vi "simflight-2.0.vi"() -> ()   [LabVIEW 2014]
uses:
  state space loop data.ctl
  <vilib>/addons/Control Design/_Model Construction/Data Typedefs.llb/CD MIMO Time Response Data.ctl
  <vilib>/addons/Control Design/_Model Construction/Data Typedefs.llb/CD Plot Types Enum.ctl
  <vilib>/Utility/miscctls.llb/LV3DPointTypeDef.ctl
  <vilib>/addons/Control Design/_Model Construction/Model Creation.llb/Model Creation SubVI/cd_Create State Space Model.vi
  <vilib>/Utility/inputDevices.llb/joystickAcquire.vi
  Data Xfer/subvis/Curcular Buffer Data History.vi
  <vilib>/addons/Control Design/_Time Response Analysis/Time Response.llb/Time Response subVI/cd_Linear Simulation (State-Space).vi
  <vilib>/addons/Control Design/_Model Construction/NI_LinSys_Model Creation.lvlib
  <vilib>/addons/Control Design/_Time Response Analysis/NI_CD_Time Response.lvlib
  <vilib>/addons/Control Design/_Model Construction/NI_LinSys_Data Typedefs.lvlib
  attitude indicator/lv-attitudecontrol.lvlib
panel:
  in  "Attitude Indicator":refnum<vi>(3d-picture)
  out "Airspeed (ft/s)":dbl(knob)=74.91519927978516 scale=0.0..120.0 scale format="%#.4f"
  out "motor (BHP)":dbl(slide) scale=-0.2..0.2
  out "altitude":T1(graph)
  out "ground track":cluster{"Time Stamp":dbl, "Data Value":dbl}[](graph)
  out "roll":dbl(slide) scale=-90.0..90.0
  out "pitch":dbl(slide) scale=-90.0..90.0
  out "rudder":dbl(slide) scale=-10.0..10.0
  out "aileron":dbl(slide) scale=-10.0..10.0
  out "elevator":dbl(slide) scale=-10.0..10.0
  out "Heading":T2(graph)={"X"=[{"Y"=[21.620706805998168, 20.15124367946963, 12.465582235692763, 7.946576972490323, 11.656565240893995, 3.970903792227472, 5.440366929130449, 13.126028372052978, 19.003880895383112, 16.244982298473555, 16.832767550897515, 24.922937499080067, 24.33515224168201, 19.81289788882929, 13.93504536742159, 21.620706805998168], "Y"=[7.099604990531346, 5.077062500919932, 10.661022401488875, 5.291796067500631, 11.248807654089271, 16.832767550897515, 18.855310035128806, 13.271350139939326, 21.36152008350073, 25.220079209877188, 26.02909620777253, 20.151243679469633, 19.34222668734553, 20.773734831883043, 12.683564887248515, 7.099604990531346]}], "z"=[{"Y"=[15.0, 16.30733614, 17.60472267, 17.43107449, 17.60472267, 18.88228568, 20.13030215, 19.78828201, 20.13030215, 21.33927393, 22.5, 22.0, 22.5, 23.60364655, 24.64181415, 23.99902654, 24.64181415, 25.60660172, 26.49066665, 25.7246222, 26.49066665, 27.28728066, 27.99038106, 27.12435565, 27.99038106, 28.59461681, 29.09538931, 28.15569669, 29.09538931, 29.48888739, 29.7721163, 28.78730854, 29.7721163, 29.94292047, 30.0, 28.5, 30.0, 29.94292047, 29.7721163, 28.78730854, 29.7721163, 29.48888739, 29.09538931, 28.15569669, 29.09538931, 28.59461681, 27.99038106, 27.12435565, 27.99038106, 27.28728066, 26.49066665, 25.7246222, 26.49066665, 25.60660172, 24.64181415, 23.99902654, 24.64181415, 23.60364655, 22.5, 22.0, 22.5, 21.33927393, 20.13030215, 19.78828201, 20.13030215, 18.88228568, 17.60472267, 17.43107449, 17.60472267, 16.30733614, 15.0, 15.0, 15.0, 13.69266386, 12.39527733, 12.56892551, 12.39527733, 11.11771432, 9.86969785, 10.21171799, 9.86969785, 8.660726074, 7.5, 8.0, 7.5, 6.396353455, 5.358185855, 6.000973464, 5.358185855, 4.393398282, 3.509333353, 4.275377796, 3.509333353, 2.712719336, 2.009618943, 2.875644347, 2.009618943, 1.405383194, 0.904610688, 1.844303309, 0.904610688, 0.511112606, 0.227883705, 1.212691458, 0.227883705, 0.057079529, 0.0, 1.5, 0.0, 0.057079529, 0.227883705, 1.212691458, 0.227883705, 0.511112606, 0.904610688, 1.844303309, 0.904610688, 1.405383194, 2.009618943, 2.875644347, 2.009618943, 2.712719336, 3.509333353, 4.275377796, 3.509333353, 4.393398282, 5.358185855, 6.000973464, 5.358185855, 6.396353455, 7.5, 8.0, 7.5, 8.660726074, 9.86969785, 10.21171799, 9.86969785, 11.11771432, 12.39527733, 12.56892551, 12.39527733, 13.69266386, 15.0, 15.0], "Y"=[30.0, 29.94292047, 29.7721163, 28.78730854, 29.7721163, 29.48888739, 29.09538931, 28.15569669, 29.09538931, 28.59461681, 27.99038106, 27.12435565, 27.99038106, 27.28728066, 26.49066665, 25.7246222, 26.49066665, 25.60660172, 24.64181415, 23.99902654, 24.64181415, 23.60364655, 22.5, 22.0, 22.5, 21.33927393, 20.13030215, 19.78828201, 20.13030215, 18.88228568, 17.60472267, 17.43107449, 17.60472267, 16.30733614, 15.0, 15.0, 15.0, 13.69266386, 12.39527733, 12.56892551, 12.39527733, 11.11771432, 9.86969785, 10.21171799, 9.86969785, 8.660726074, 7.5, 8.0, 7.5, 6.396353455, 5.358185855, 6.000973464, 5.358185855, 4.393398282, 3.509333353, 4.275377796, 3.509333353, 2.712719336, 2.009618943, 2.875644347, 2.009618943, 1.405383194, 0.904610688, 1.844303309, 0.904610688, 0.511112606, 0.227883705, 1.212691458, 0.227883705, 0.057079529, 0.0, 1.5, 0.0, 0.057079529, 0.227883705, 1.212691458, 0.227883705, 0.511112606, 0.904610688, 1.844303309, 0.904610688, 1.405383194, 2.009618943, 2.875644347, 2.009618943, 2.712719336, 3.509333353, 4.275377796, 3.509333353, 4.393398282, 5.358185855, 6.000973464, 5.358185855, 6.396353455, 7.5, 8.0, 7.5, 8.660726074, 9.86969785, 10.21171799, 9.86969785, 11.11771432, 12.39527733, 12.56892551, 12.39527733, 13.69266386, 15.0, 15.0, 15.0, 16.30733614, 17.60472267, 17.43107449, 17.60472267, 18.88228568, 20.13030215, 19.78828201, 20.13030215, 21.33927393, 22.5, 22.0, 22.5, 23.60364655, 24.64181415, 23.99902654, 24.64181415, 25.60660172, 26.49066665, 25.7246222, 26.49066665, 27.28728066, 27.99038106, 27.12435565, 27.99038106, 28.59461681, 29.09538931, 28.15569669, 29.09538931, 29.48888739, 29.7721163, 28.78730854, 29.7721163, 29.94292047, 30.0, 28.5]}]}
  in  "visual":refnum<k7>(container) caption="3D 파라미터형 표면"
  in  "stop":bool
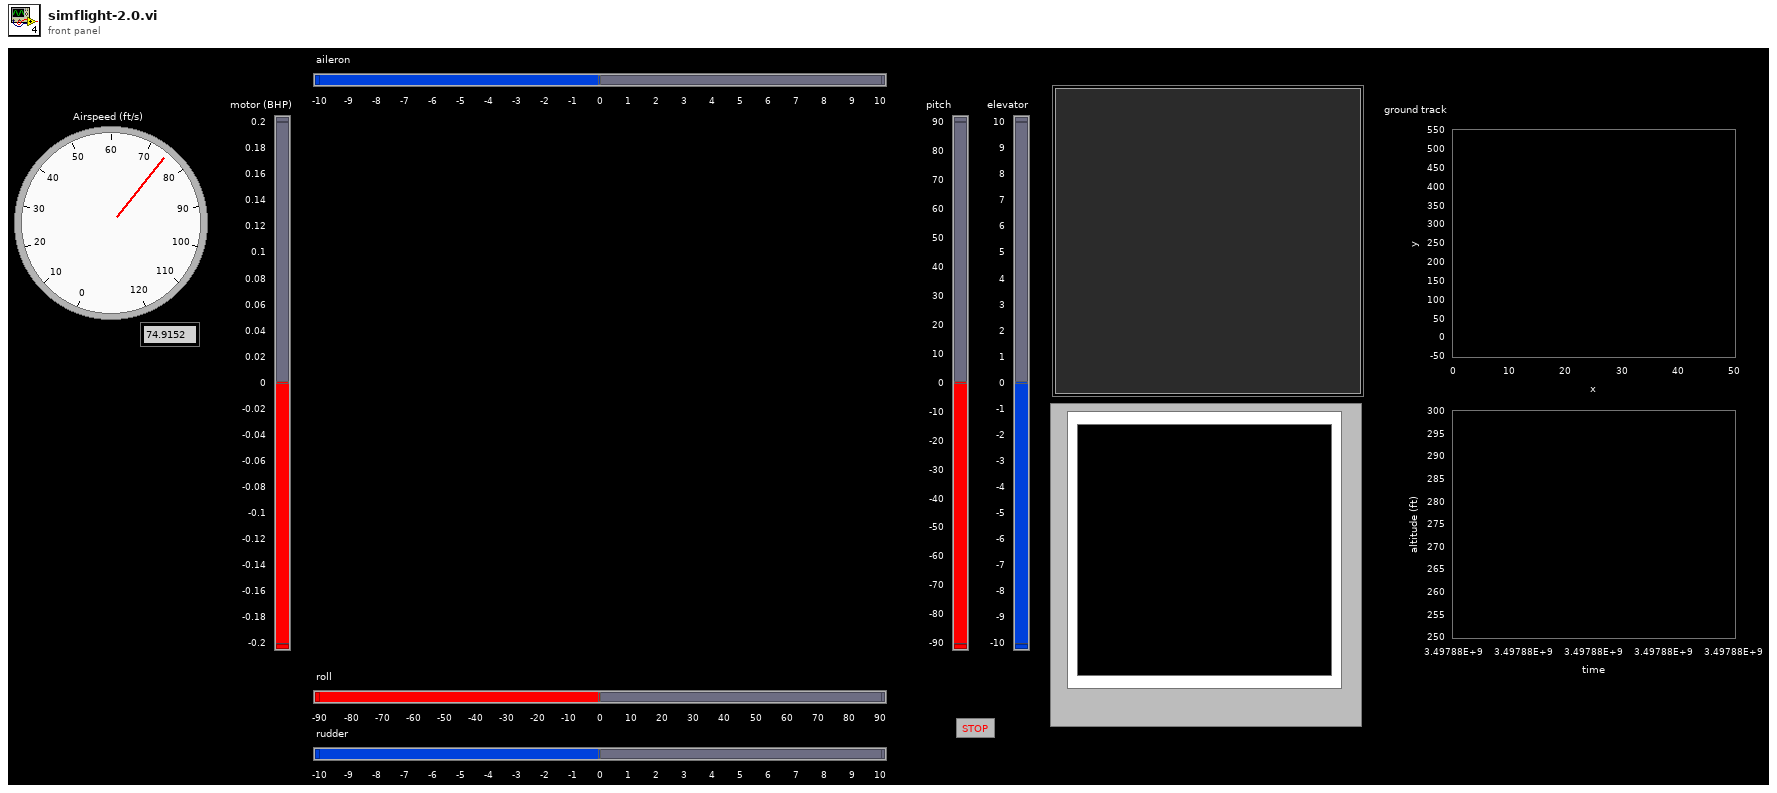
[diagram p1: front panel]
types:
  T1 = cluster{cluster{"Time Stamp":dbl, "Data Value":dbl}[]}[]
  T2 = cluster{"X":cluster{"Y":dbl[], "Y":dbl[]}[], "z":cluster{"Y":dbl[], "Y":dbl[]}[]}
  T3 = typedef "state space loop data.ctl" = cluster{"d_elevator (rad)":dbl, "d_rudder (rad)":dbl, "d_aileron (rad)":dbl, "d_motor (bhp)":dbl, "loop start (s)":dbl, "dT":dbl, "time now":dbl, "Sim Data":T4, "sim conditions":dbl[], "timestamp":dbl}
  T4 = typedef "NI_LinSys_Data Typedefs.lvlib/CD MIMO Time Response Data.ctl" = cluster{"Time":dbl[], "Outputs Data":dbl[][][], "States Data":dbl[][][], "plot type":T5}
  T5 = typedef "NI_LinSys_Data Typedefs.lvlib/CD Plot Types Enum.ctl" = enum16{"bode-magnitude", "bode-phase", "nichols", "nyquist", "singular values", "step", "impulse", "initial", "simulation", "nyquist with separation"}
  T6 = typedef "NI_LinSys_Model Typedefs.lvlib/CD State Space Model (MIMO).ctl" = cluster{"properties":T7, "A":dbl[][], "B":dbl[][], "C":dbl[][], "D":dbl[][], "StateNames":string[], "Transport Delay":dbl[][]}
  T7 = typedef "NI_LinSys_Model Typedefs.lvlib/CD General Elements.ctl" = cluster{"Model name":string, "Input names":string[], "Output names":string[], "Input Delays":dbl[], "Output Delays":dbl[], "Sampling Time":dbl, "Notes":string}
  T8 = typedef "lv-attitudecontrol.lvlib/AttitudeHandle.ctl" = cluster{"First Scene Object":refnum<vi>, "Drum":refnum<vi>, "Window":refnum<vi>, "Dial":refnum<vi>, "Scene Graph":refnum<vi>, "Last Drum Pitch":dbl, "Last Drum Roll ":dbl, "Last Dial Roll":dbl}
  T9 = cluster{"X axis":i32, "Y axis":i32, "Z axis":i32, "X axis rotation":i32, "Y axis rotation":i32, "Z axis rotation":i32, "U axis":i32, "V axis":i32}
  T10 = typedef "LV3DPointTypeDef.ctl" = cluster{"X":sgl, "Y":sgl, "Z":sgl}
  T11 = cluster{cluster{"Time Stamp":dbl, "Data Value":dbl}[]}
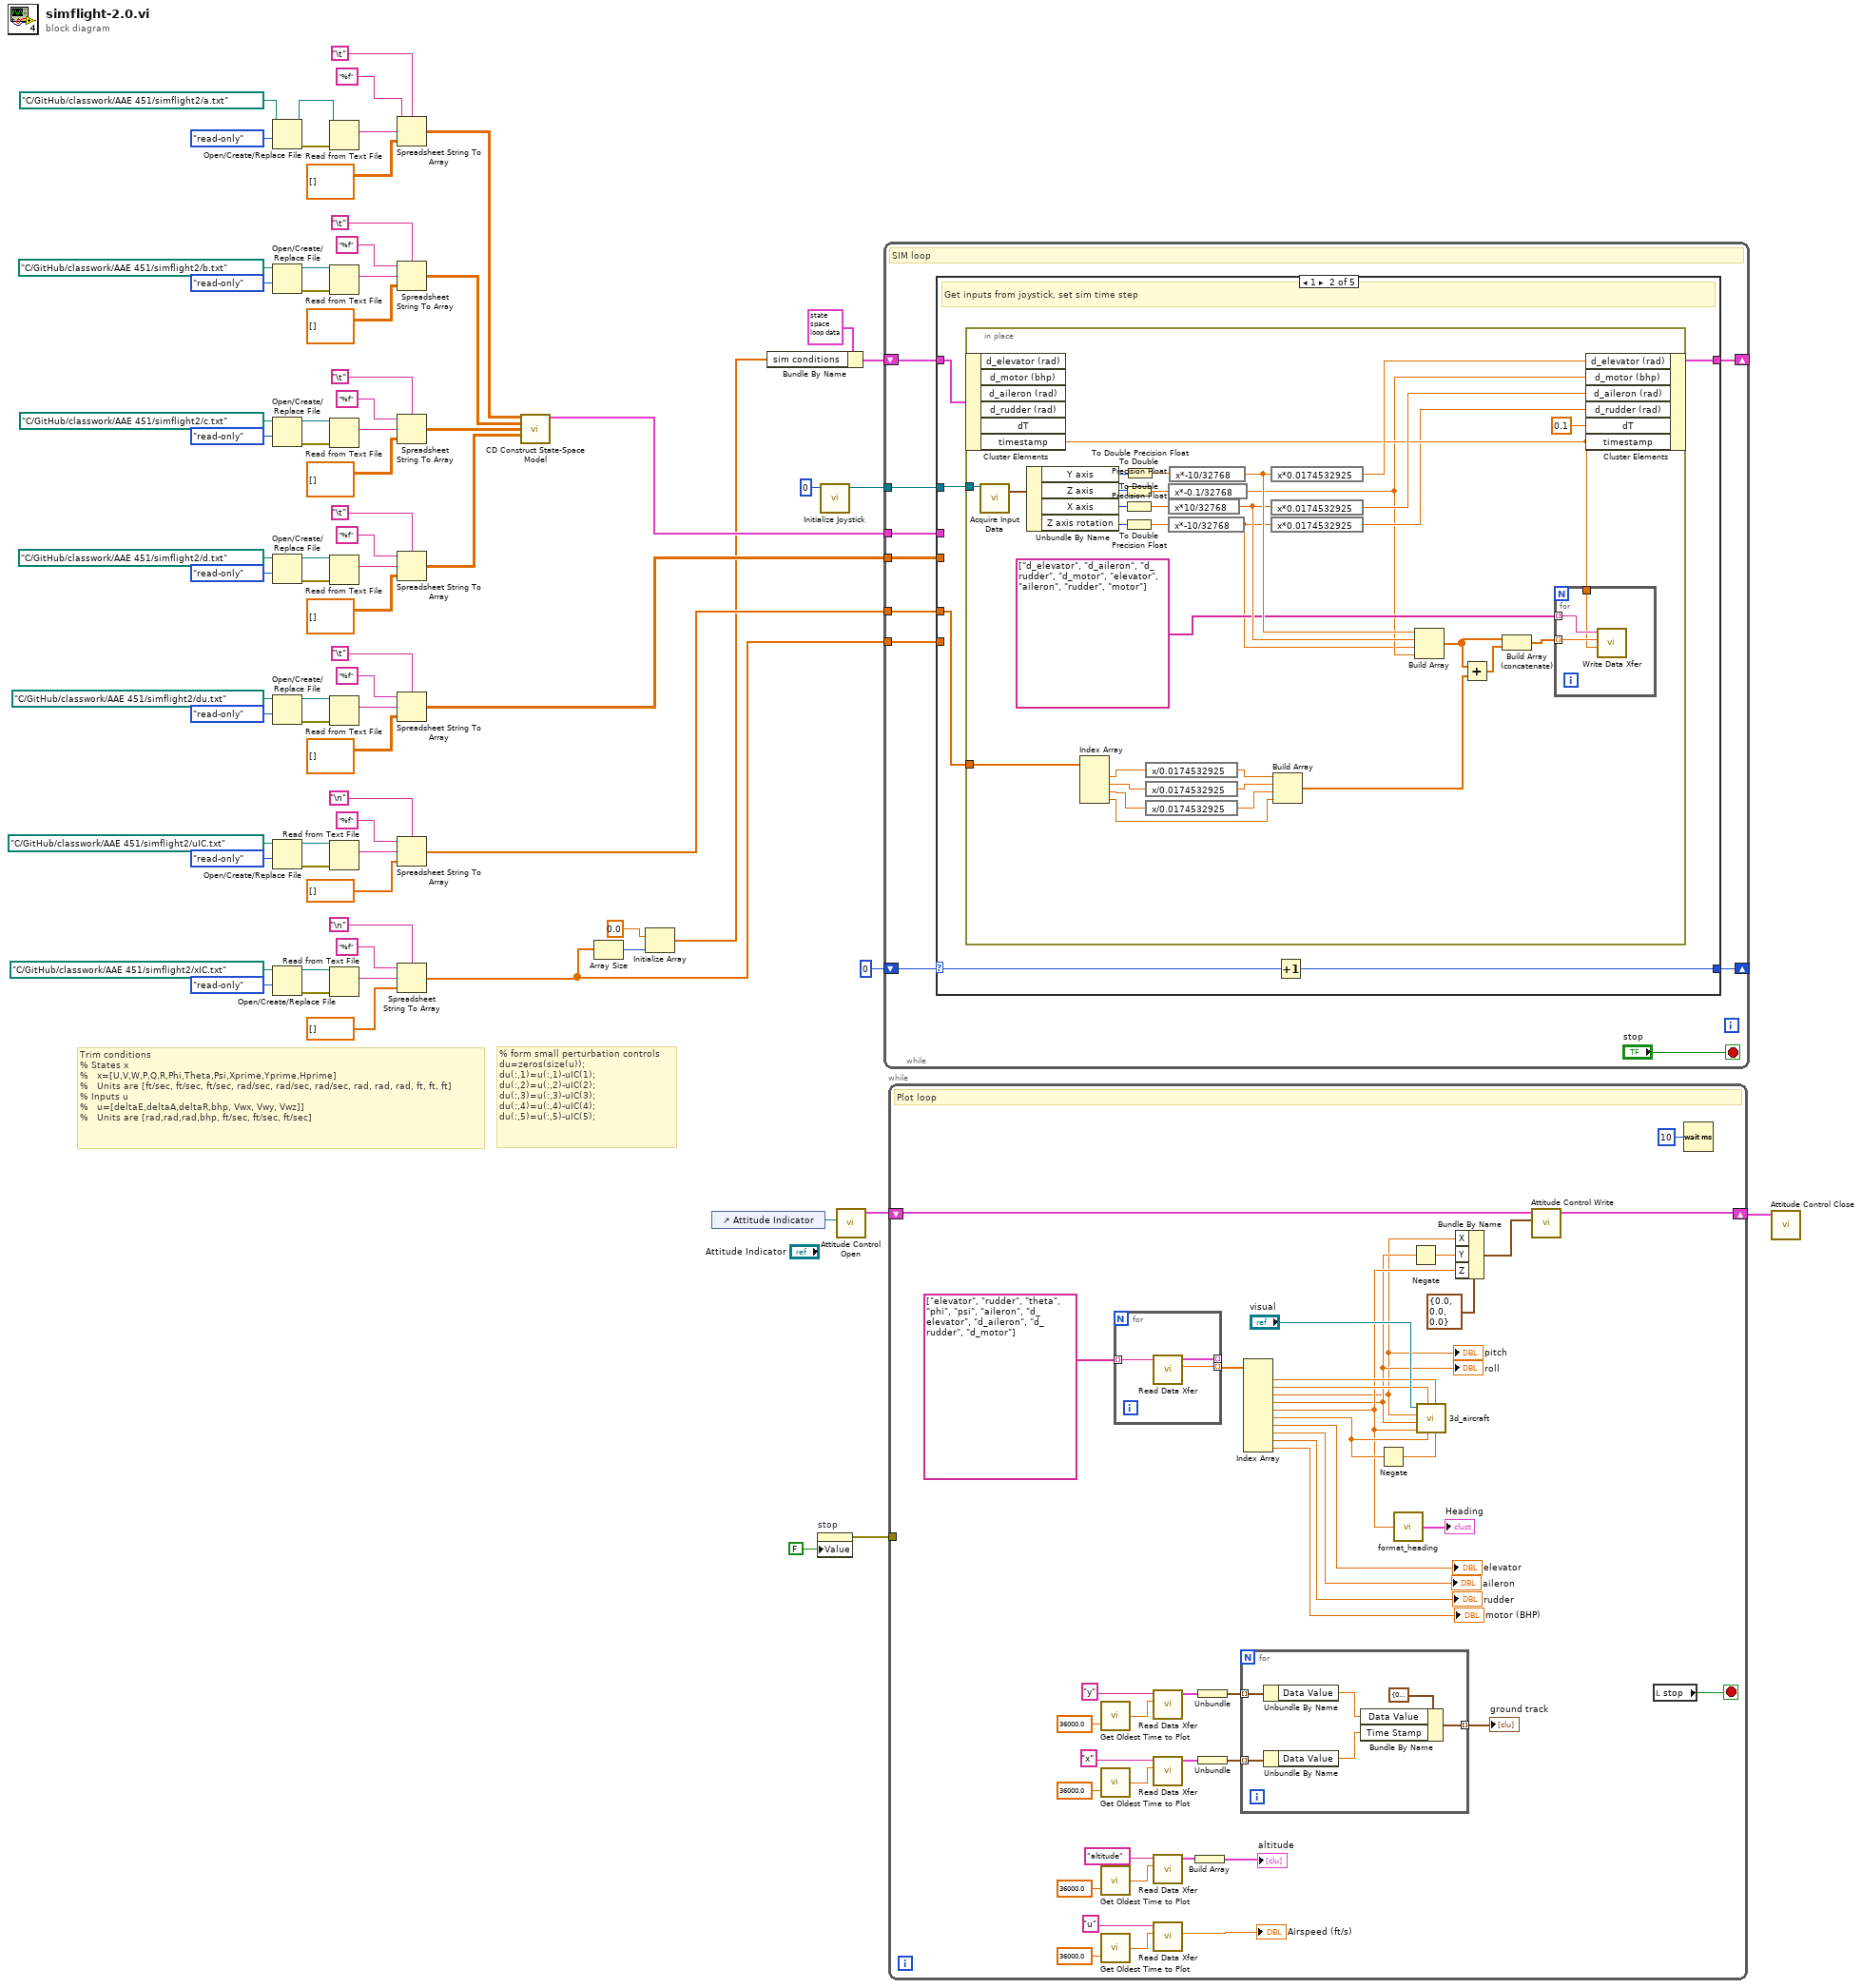
[diagram p0: block diagram]
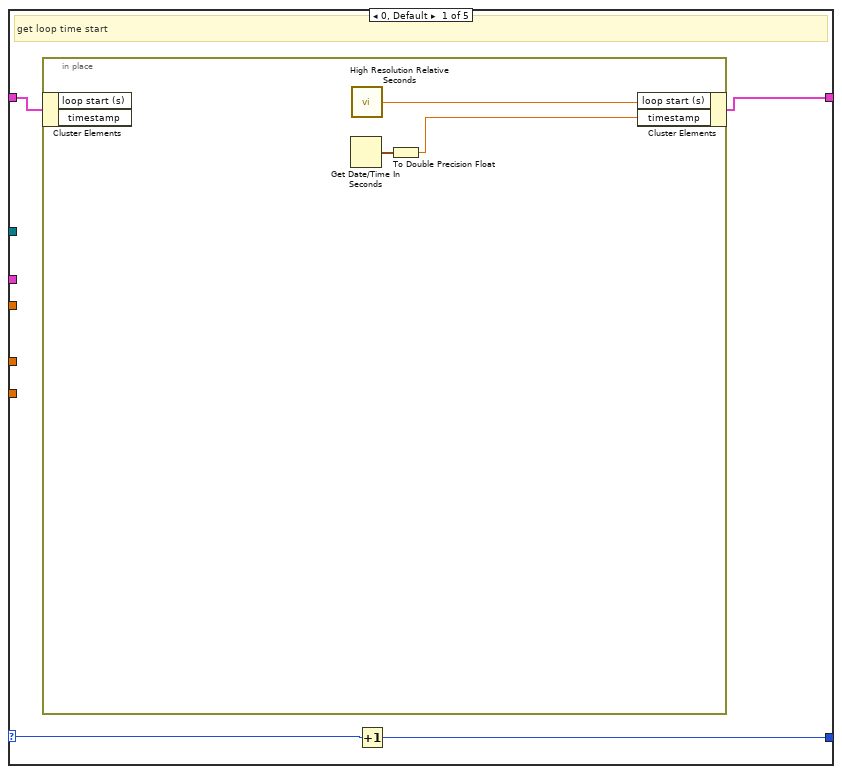
[diagram p2: hidden frame]
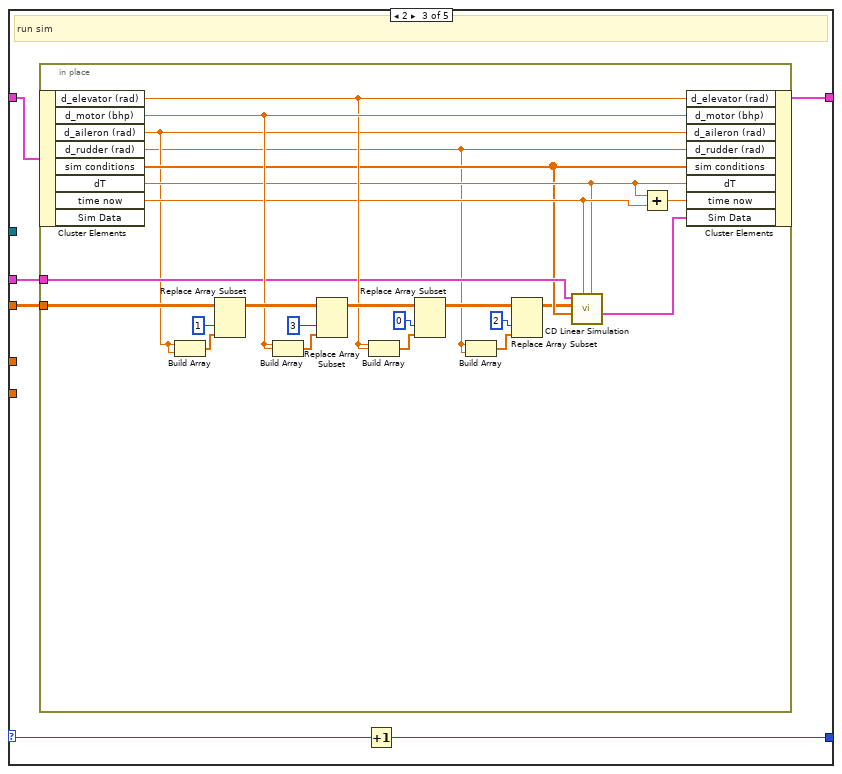
[diagram p3: hidden frame]
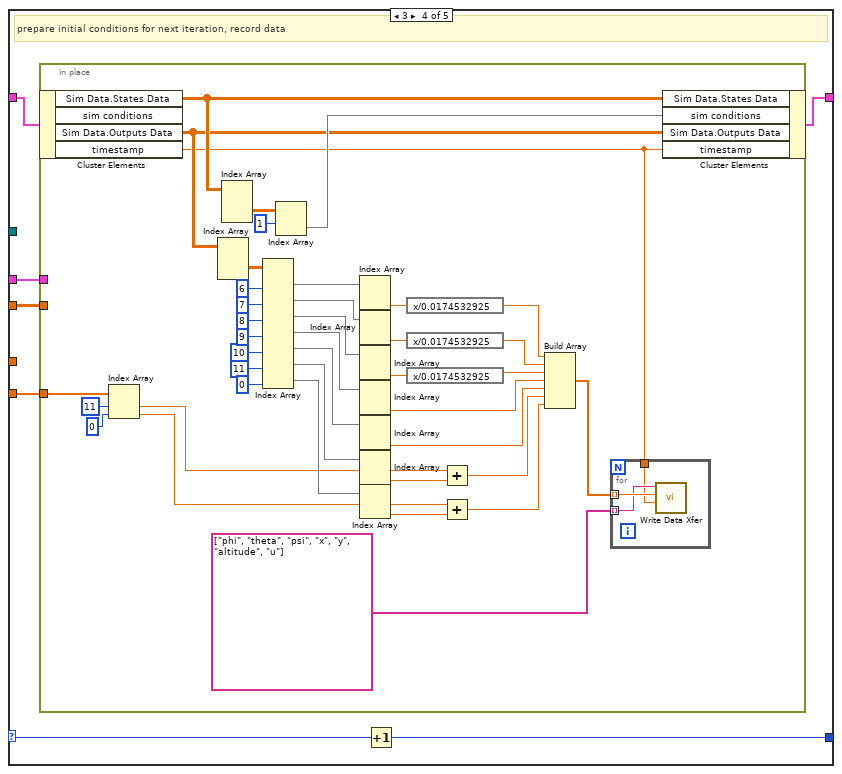
[diagram p4: hidden frame]
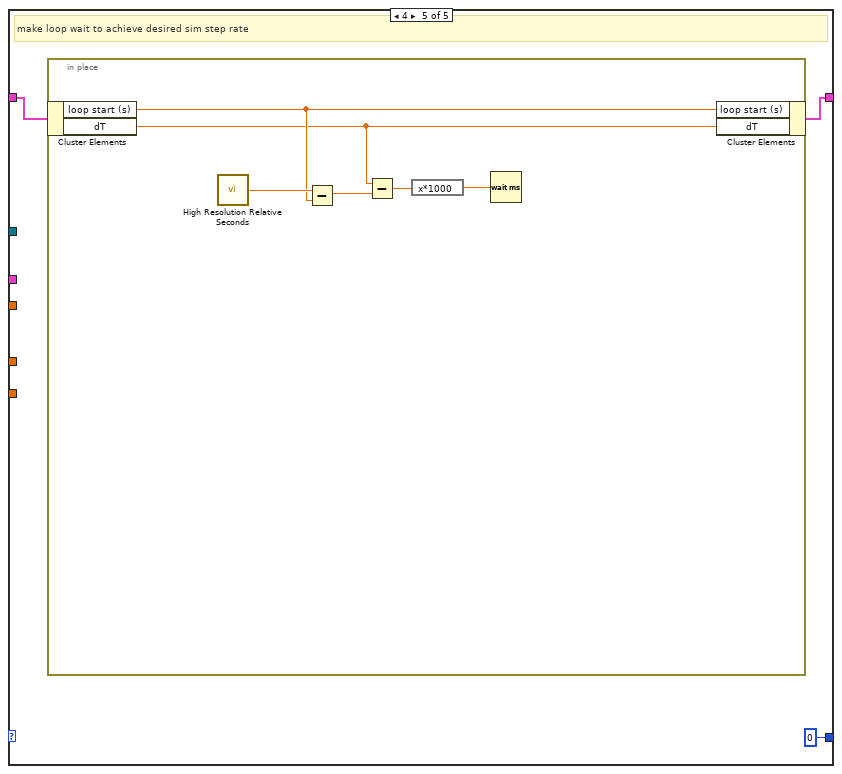
[diagram p5: hidden frame]
diagram:
  # "% form small perturbation controls\ndu=zeros(size(u));\ndu(:,1)=u(:,1)-uIC(1);\ndu(:,2)=u(:,2)-uIC(2);\ndu(:,3)=u(:,3)-uIC(3);\ndu(:,4)=u(:,4)-uIC(4);\ndu(:,5)=u(:,5)-uIC(5);"
  # "Trim conditions\n% States x\n%   x=[U,V,W,P,Q,R,Phi,Theta,Psi,Xprime,Yprime,Hprime]\n%   Units are [ft/sec, ft/sec, ft/sec, rad/sec, rad/sec, rad/sec, rad, rad, rad, ft, ft, ft]\n% Inputs u\n%   u=[deltaE,deltaA,deltaR,bhp, Vwx, Vwy, Vwz]]\n%   Units are [rad,rad,rad,bhp, ft/sec, ft/sec, ft/sec]"
  n1 = Open/Create/Replace File(file path (use dialog)=path "C:/GitHub/classwork/AAE 451/simflight2/a.txt", access (0:read/write)=enum16{"read/write", "read-only", "write-only"}."read-only") -> (refnum out=w74:refnum<file>, error out=w75:errorcluster)  [unwired: 4 in, 1 out]
  n2 = Open/Create/Replace File(file path (use dialog)=path "C:/GitHub/classwork/AAE 451/simflight2/b.txt", access (0:read/write)=enum16{"read/write", "read-only", "write-only"}."read-only") -> (refnum out=w65:refnum<file>, error out=w64:errorcluster)  [unwired: 4 in, 1 out]
  n3 = Open/Create/Replace File(file path (use dialog)=path "C:/GitHub/classwork/AAE 451/simflight2/c.txt", access (0:read/write)=enum16{"read/write", "read-only", "write-only"}."read-only") -> (refnum out=w58:refnum<file>, error out=w59:errorcluster)  [unwired: 4 in, 1 out]
  n4 = Open/Create/Replace File(file path (use dialog)=path "C:/GitHub/classwork/AAE 451/simflight2/d.txt", access (0:read/write)=enum16{"read/write", "read-only", "write-only"}."read-only") -> (refnum out=w49:refnum<file>, error out=w48:errorcluster)  [unwired: 4 in, 1 out]
  n5 = Open/Create/Replace File(file path (use dialog)=path "C:/GitHub/classwork/AAE 451/simflight2/du.txt", access (0:read/write)=enum16{"read/write", "read-only", "write-only"}."read-only") -> (refnum out=w38:refnum<file>, error out=w39:errorcluster)  [unwired: 4 in, 1 out]
  n6 = Open/Create/Replace File(file path (use dialog)=path "C:/GitHub/classwork/AAE 451/simflight2/uIC.txt", access (0:read/write)=enum16{"read/write", "read-only", "write-only"}."read-only") -> (refnum out=w15:refnum<file>, error out=w16:errorcluster)  [unwired: 4 in, 1 out]
  n7 = Open/Create/Replace File(file path (use dialog)=path "C:/GitHub/classwork/AAE 451/simflight2/xIC.txt", access (0:read/write)=enum16{"read/write", "read-only", "write-only"}."read-only") -> (refnum out=w30:refnum<file>, error out=w31:errorcluster)  [unwired: 4 in, 1 out]
  n8 = Read from Text File(file (use dialog)=w74, error in=w75) -> (text=w73:string)  [unwired: 2 in, 3 out]
  n9 = Read from Text File(file (use dialog)=w65, error in=w64) -> (text=w66:string)  [unwired: 2 in, 3 out]
  n10 = Read from Text File(file (use dialog)=w58, error in=w59) -> (text=w57:string)  [unwired: 2 in, 3 out]
  n11 = Read from Text File(file (use dialog)=w49, error in=w48) -> (text=w50:string)  [unwired: 2 in, 3 out]
  n12 = Read from Text File(file (use dialog)=w38, error in=w39) -> (text=w37:string)  [unwired: 2 in, 3 out]
  n13 = Read from Text File(file (use dialog)=w15, error in=w16) -> (text=w14:string)  [unwired: 2 in, 3 out]
  n14 = Read from Text File(file (use dialog)=w30, error in=w31) -> (text=w29:string)  [unwired: 2 in, 3 out]
  n15 = Spreadsheet String To Array(delimiter (Tab)="\t", format string="%f", spreadsheet string=w73, array type (2D Dbl)=dbl[][] []) -> (array=w45:dbl[][])
  n16 = Spreadsheet String To Array(delimiter (Tab)="\t", format string="%f", spreadsheet string=w66, array type (2D Dbl)=dbl[][] []) -> (array=w44:dbl[][])
  n17 = Spreadsheet String To Array(delimiter (Tab)="\t", format string="%f", spreadsheet string=w57, array type (2D Dbl)=dbl[][] []) -> (array=w42:dbl[][])
  n18 = Spreadsheet String To Array(delimiter (Tab)="\t", format string="%f", spreadsheet string=w50, array type (2D Dbl)=dbl[][] []) -> (array=w43:dbl[][])
  n19 = Spreadsheet String To Array(delimiter (Tab)="\t", format string="%f", spreadsheet string=w37, array type (2D Dbl)=dbl[][] []) -> (array=w21:dbl[][])
  n20 = Spreadsheet String To Array(delimiter (Tab)="\n", format string="%f", spreadsheet string=w14, array type (2D Dbl)=dbl[] []) -> (array=w10:dbl[])
  n21 = Spreadsheet String To Array(delimiter (Tab)="\n", format string="%f", spreadsheet string=w29, array type (2D Dbl)=dbl[] []) -> (array=w4:dbl[])
  n22 = call-poly <vilib>:"CD Construct State-Space Model.vi"("A"=w45, "B"=w44, "C"=w42, "D"=w43) -> ("State-Space Model"=w22:T6)  [unwired: 10 in, 1 out]
  n23 = Array Size(array=w4) -> (size(s)=w7:i32)
  n24 = Initialize Array(0.0, w7) -> (w5:dbl[])
  n25 = control-ref of="Attitude Indicator"() -> (w3:refnum<vi>)
  n26 = Bundle By Name(cluster=T3 {"d_elevator (rad)"=0.0, "d_rudder (rad)"=0.0, "d_aileron (rad)"=0.0, "d_motor (bhp)"=0.0, "loop start (s)"=0.0, "dT"=0.0, "time now"=0.0, "Sim Data"={"Time"=[], "Outputs Data"=[], "States Data"=[], "plot type"=enum."step"}, "sim conditions"=[], "timestamp"=0.0}, "sim conditions"=w5) -> (w19:T3)
  n27 = property on="stop" class="Bool (strict)"("Value"=FALSE ("stop")) -> (error out=w8:errorcluster)  [unwired: 2 in, 1 out]
  n28 = call <vilib>:"Initialize Joystick.vi"("device index"=0) -> ("device ID"=w24:refnum<k1>)  [unwired: 9 in, 1 out]
  n29 = call "Attitude Control Open.vi"("Scene Graph"=w3) -> ("Attitude Control Handle"=w2:T8)  [unwired: 9 in, 1 out]
  n30 = while {
    shift-right: [w86] -> _
    shift-left: w19 -> [w87]
    tunnel: w24 -> [w85]
    shift-right: [w84] -> _
    shift-left: 0 -> [w83]
    tunnel: w22 -> [w81]
    tunnel: w21 -> [w80]
    tunnel: w10 -> [w79]
    tunnel: w4 -> [w78]
    stop <- "stop" stop-if-true
    # "SIM loop"
    n31 = case shown="1" w83 {
      tunnel: w87 -> [w89 w99 w141 w171 w216]
      tunnel: [w88 w98 w140 w170 w215] -> w86
      tunnel: w85 -> [_ w100 _ _ _]
      selector: w83 -> [w91 w97 w139 w169 _]
      tunnel: [w90 w96 w138 w168 0] -> w84
      tunnel: w81 -> [_ _ w136 w166 _]
      tunnel: w80 -> [_ _ w137 w167 _]
      tunnel: w79 -> [_ w95 _ _ _]
      tunnel: w78 -> [_ _ _ w165 _]
      frame 0, Default {
        # "get loop time start"
        n32 = in-place {
          n33 = in-place-cluster #1(w89) -> ()  [unwired: 2 out]
          n34 = Get Date/Time In Seconds() -> (seconds since 1Jan1904=w93:timestamp)
          n35 = call <vilib>:"High Resolution Relative Seconds.vi"() -> ("relative seconds"=w94:dbl)
          n36 = To Double Precision Float(number=w93) -> (double precision float=w92:dbl)
          n37 = in-place-cluster #1("loop start (s)"=w94, "timestamp"=w92) -> (w88:T3)
        }
        n38 = Increment(x=w91) -> (x+1=w90:i32)
      }
      frame 1 {
        # "Get inputs from joystick, set sim time step"
        n39 = in-place {
          in-place-border: w100 -> [w130]
          in-place-border: w95 -> [w118]
          n40 = in-place-cluster #2(w99) -> ("timestamp"=w119:dbl)  [unwired: 5 out]
          n41 = call-poly <vilib>:"Acquire Input Data.vi"("device ID"=w130) -> ("axis info"=w129:T9)  [unwired: 14 in, 4 out]
          n42 = Unbundle By Name(w129) -> ("Y axis"=w131:i32, "Z axis"=w126:i32, "X axis"=w125:i32, "Z axis rotation"=w108:i32)
          n43 = Index Array(array=w118) -> (element #1=w113:dbl, element #2=w111:dbl, element #3=w103:dbl, element #4=w101:dbl)  [unwired: 4 in]
          n44 = To Double Precision Float(number=w126) -> (double precision float=w127:dbl)
          n45 = To Double Precision Float(number=w125) -> (double precision float=w109:dbl)
          n46 = To Double Precision Float(number=w108) -> (double precision float=w107:dbl)
          n47 = To Double Precision Float(number=w131) -> (double precision float=w132:dbl)
          n48 = expression code="x/0.0174532925"(w113) -> (w112:dbl)
          n49 = expression code="x/0.0174532925"(w111) -> (w110:dbl)
          n50 = expression code="x/0.0174532925"(w103) -> (w102:dbl)
          n51 = expression code="x*-0.1/32768"(w127) -> (w105:dbl)
          n52 = expression code="x*10/32768"(w109) -> (w121:dbl)
          n53 = expression code="x*-10/32768"(w107) -> (w104:dbl)
          n54 = expression code="x*-10/32768"(w132) -> (w122:dbl)
          n55 = expression code="x*0.0174532925"(w122) -> (w128:dbl)
          n56 = expression code="x*0.0174532925"(w121) -> (w124:dbl)
          n57 = expression code="x*0.0174532925"(w104) -> (w106:dbl)
          n58 = Build Array(w112, w110, w102, w101) -> (w117:dbl[])
          n59 = Build Array(w122, w121, w104, w105) -> (w115:dbl[])
          n60 = Add(x=w115, y=w117) -> (x+y=w116:dbl[])
          n61 = Build Array (concatenate)(w115, w116) -> (w114:dbl[])
          n62 = for {
            tunnel: w114 -> [w135] mode=indexing
            tunnel: string[] ["d_elevator", "d_aileron", "d_rudder", "d_motor", "elevator", "aileron", "rudder", "motor"] -> [w134] mode=indexing
            tunnel: w119 -> [w133]
            n63 = call "Write Data Xfer.vi"("Time Stamp"=w133, "Data Value"=w135, "Device Name"=w134) -> ()  [unwired: 8 in, 1 out]
          }
          n64 = in-place-cluster #2("d_elevator (rad)"=w128, "d_motor (bhp)"=w105, "d_aileron (rad)"=w124, "d_rudder (rad)"=w106, "dT"=0.1, "timestamp"=w119) -> (w98:T3)
        }
        n65 = Increment(x=w97) -> (x+1=w96:i32)
      }
      frame 2 {
        # "run sim"
        n66 = in-place {
          in-place-border: w137 -> [w159]
          in-place-border: w136 -> [w153]
          n67 = in-place-cluster #3(w141) -> ("d_elevator (rad)"=w154:dbl, "d_motor (bhp)"=w156:dbl, "d_aileron (rad)"=w147:dbl, "d_rudder (rad)"=w142:dbl, "sim conditions"=w148:dbl[], "dT"=w151:dbl, "time now"=w152:dbl)  [unwired: 1 out]
          n68 = Build Array(w147, w147) -> (w158:dbl[])
          n69 = Replace Array Subset(array=w159, new element=w158, index (col)=1 ("disabled index (col)")) -> (w164:dbl[][])  [unwired: 1 in]
          n70 = Build Array(w156, w156) -> (w157:dbl[])
          n71 = Replace Array Subset(array=w164, new element=w157, index (col)=3 ("disabled index (col)")) -> (w161:dbl[][])  [unwired: 1 in]
          n72 = Build Array(w154, w154) -> (w155:dbl[])
          n73 = Replace Array Subset(array=w161, new element=w155, index (col)=0 ("index")) -> (w144:dbl[][])  [unwired: 1 in]
          n74 = Build Array(w142, w142) -> (w146:dbl[])
          n75 = Replace Array Subset(array=w144, new element=w146, index (col)=2 ("index")) -> (w143:dbl[][])  [unwired: 1 in]
          n76 = call-poly <vilib>:"CD Linear Simulation.vi"("Delta t"=w151, "Initial Time"=w152, "Initial Conditions"=w148, "Inputs"=w143, "State-Space Model"=w153) -> ("Simulation Data"=w149:T4)  [unwired: 3 in, 3 out]
          n77 = Add(x=w151, y=w152) -> (x+y=w150:dbl)
          n78 = in-place-cluster #3("d_elevator (rad)"=w154, "d_motor (bhp)"=w156, "d_aileron (rad)"=w147, "d_rudder (rad)"=w142, "sim conditions"=w148, "dT"=w151, "time now"=w150, "Sim Data"=w149) -> (w140:T3)
        }
        n79 = Increment(x=w139) -> (x+1=w138:i32)
      }
      frame 3 {
        # "prepare initial conditions for next iteration, record data"
        n80 = in-place {
          in-place-border: w167 -> [_]
          in-place-border: w166 -> [_]
          in-place-border: w165 -> [w180]
          n81 = in-place-cluster #4(w171) -> ("Sim Data.States Data"=w209:dbl[][][], "Sim Data.Outputs Data"=w207:dbl[][][], "timestamp"=w190:dbl)  [unwired: 1 out]
          n82 = Index Array(array=w180, index #1=11 ("index"), index #2=0 ("index")) -> (element #1=w178:dbl, element #2=w173:dbl)
          n83 = Index Array(array=w207) -> (element=w206:dbl[][])  [unwired: 3 in]
          n84 = Index Array(array=w209) -> (element=w210:dbl[][])  [unwired: 3 in]
          n85 = Index Array(array=w206, index (col) #1=6 ("disabled index (col)"), index (col) #2=7 ("disabled index (col)"), index (col) #3=8 ("disabled index (col)"), index (col) #4=9 ("disabled index (col)"), index (col) #5=10 ("disabled index (col)"), index (col) #6=11 ("disabled index (col)"), index (col) #7=0 ("disabled index (col)")) -> (element #1=w204:dbl[], element #2=w203:dbl[], element #3=w202:dbl[], element #4=w201:dbl[], element #5=w200:dbl[], element #6=w199:dbl[], element #7=w181:dbl[])  [unwired: 7 in]
          n86 = Index Array(array=w210, index (row)=1) -> (element=w208:dbl[])  [unwired: 1 in]
          n87 = Index Array(array=w204) -> (element #2=w198:dbl)  [unwired: 2 in, 1 out]
          n88 = Index Array(array=w203) -> (element #2=w195:dbl)  [unwired: 2 in, 1 out]
          n89 = Index Array(array=w202) -> (element #2=w194:dbl)  [unwired: 2 in, 1 out]
          n90 = Index Array(array=w201) -> (element #2=w186:dbl)  [unwired: 2 in, 1 out]
          n91 = Index Array(array=w200) -> (element #2=w185:dbl)  [unwired: 2 in, 1 out]
          n92 = Index Array(array=w199) -> (element #2=w179:dbl)  [unwired: 2 in, 1 out]
          n93 = Index Array(array=w181) -> (element #2=w174:dbl)  [unwired: 2 in, 1 out]
          n94 = expression code="x/0.0174532925"(w198) -> (w189:dbl)
          n95 = expression code="x/0.0174532925"(w195) -> (w188:dbl)
          n96 = expression code="x/0.0174532925"(w194) -> (w187:dbl)
          n97 = Add(x=w178, y=w179) -> (x+y=w175:dbl)
          n98 = Add(x=w173, y=w174) -> (x+y=w172:dbl)
          n99 = Build Array(w189, w188, w187, w186, w185, w175, w172) -> (w184:dbl[])
          n100 = for {
            tunnel: w184 -> [w214] mode=indexing
            tunnel: string[] ["phi", "theta", "psi", "x", "y", "altitude", "u"] -> [w213] mode=indexing
            tunnel: w190 -> [w212]
            n101 = call "Write Data Xfer.vi"("Time Stamp"=w212, "Data Value"=w214, "Device Name"=w213) -> ()  [unwired: 8 in, 1 out]
          }
          n102 = in-place-cluster #4("Sim Data.States Data"=w209, "sim conditions"=w208, "Sim Data.Outputs Data"=w207, "timestamp"=w190) -> (w170:T3)
        }
        n103 = Increment(x=w169) -> (x+1=w168:i32)
      }
      frame 4 {
        # "make loop wait to achieve desired sim step rate"
        n104 = in-place {
          n105 = in-place-cluster #5(w216) -> ("loop start (s)"=w221:dbl, "dT"=w220:dbl)
          n106 = call <vilib>:"High Resolution Relative Seconds.vi"() -> ("relative seconds"=w223:dbl)
          n107 = Subtract(x=w223, y=w221) -> (x-y=w222:dbl)
          n108 = Subtract(x=w220, y=w222) -> (x-y=w218:dbl)
          n109 = expression code="x*1000"(w218) -> (w219:dbl)
          n110 = Wait (ms)(milliseconds to wait=w219) -> ()  [unwired: 1 out]
          n111 = in-place-cluster #5("loop start (s)"=w221, "dT"=w220) -> (w215:T3)
        }
      }
    }
  }
  n112 = while {
    tunnel: w8 -> [_]
    shift-right: [w227] -> w1
    shift-left: w2 -> [w229]
    stop <- w265 stop-if-true
    # "Plot loop"
    n113 = call "Get Oldest Time to Plot.vi"("History Length"=36000.0) -> ("Oldest Time to Plot"=w250:dbl)  [unwired: 1 in]
    n114 = call "Get Oldest Time to Plot.vi"("History Length"=36000.0) -> ("Oldest Time to Plot"=w249:dbl)  [unwired: 1 in]
    n115 = call "Get Oldest Time to Plot.vi"("History Length"=36000.0) -> ("Oldest Time to Plot"=w239:dbl)  [unwired: 1 in]
    n116 = call "Get Oldest Time to Plot.vi"("History Length"=36000.0) -> ("Oldest Time to Plot"=w235:dbl)  [unwired: 1 in]
    n117 = for {
      tunnel: string[] ["elevator", "rudder", "theta", "phi", "psi", "aileron", "d_elevator", "d_aileron", "d_rudder", "d_motor"] -> [w274] mode=indexing
      tunnel: [w273] -> w261 mode=indexing
      tunnel: [w272] -> _ mode=indexing
      n118 = call "Read Data Xfer.vi"("Device Name"=w274) -> ("Latest Value"=w273:dbl, "Truncated Data History"=w272:T11)  [unwired: 7 in, 2 out]
    }
    n119 = call "Read Data Xfer.vi"("Oldest time to Plot"=w250, "Device Name"="y") -> ("Truncated Data History"=w246:T11)  [unwired: 6 in, 3 out]
    n120 = call "Read Data Xfer.vi"("Oldest time to Plot"=w249, "Device Name"="x") -> ("Truncated Data History"=w244:T11)  [unwired: 6 in, 3 out]
    n121 = call "Read Data Xfer.vi"("Oldest time to Plot"=w239, "Device Name"="altitude") -> ("Truncated Data History"=w238:T11)  [unwired: 6 in, 3 out]
    n122 = call "Read Data Xfer.vi"("Oldest time to Plot"=w235, "Device Name"="u") -> ("Latest Value"=→"Airspeed (ft/s)":dbl)  [unwired: 6 in, 3 out]
    n123 = Build Array(w238) -> (→"altitude":T1)
    n124 = Unbundle(w246) -> (w245:cluster{"Time Stamp":dbl, "Data Value":dbl}[])
    n125 = Unbundle(w244) -> (w243:cluster{"Time Stamp":dbl, "Data Value":dbl}[])
    n126 = for {
      tunnel: w245 -> [w271] mode=indexing
      tunnel: w243 -> [w270] mode=indexing
      tunnel: [w266] -> w242 mode=indexing
      n127 = Unbundle By Name(w271) -> ("Data Value"=w268:dbl)
      n128 = Unbundle By Name(w270) -> ("Data Value"=w267:dbl)
      n129 = Bundle By Name(cluster=cluster{"Time Stamp":dbl, "Data Value":dbl} {"Time Stamp"=0.0, "Data Value"=0.0}, "Data Value"=w268, "Time Stamp"=w267) -> (w266:cluster{"Time Stamp":dbl, "Data Value":dbl})
    }
    "ground track" <- w242
    n130 = Index Array(array=w261) -> (element #1=w260:dbl, element #2=w254:dbl, element #3=w224:dbl, element #4=w225:dbl, element #5=w230:dbl, element #6=w255:dbl, element #7=→"elevator":dbl, element #8=→"aileron":dbl, element #9=→"rudder":dbl, element #10=→"motor (BHP)":dbl)  [unwired: 10 in]
    "roll" <- w225
    "pitch" <- w224
    n131 = Negate(x=w255) -> (-x=w259:dbl)
    n132 = call "format_heading.vi"("Heading (deg)"=w230) -> ("heading (formatted)"=→"Heading":T2)
    n133 = Negate(x=w225) -> (-x=w226:dbl)
    n134 = call "3d_aircraft.vi"("RH Aileron"=w259, "Elevator"=w260, "LH Aileron"=w255, "Rudder"=w254, "Heading (deg)"=w230, "Roll (deg)"=w225, "Pitch (deg)"=w224, "visual"="visual") -> ()  [unwired: 4 in]
    n135 = Bundle By Name(cluster=T10 {"X"=0.0, "Y"=0.0, "Z"=0.0} ("Control 1"), "X"=w224, "Y"=w226, "Z"=w230) -> (w228:T10)
    n136 = call "Attitude Control Write.vi"("pitch (x), roll (y), yaw (z)"=w228, "Attitude Control Handle In"=w229) -> ("Attitude Control Handle Out"=w227:T8)  [unwired: 8 in, 1 out]
    n137 = local read "stop"() -> (w265:bool)
    n138 = Wait (ms)(milliseconds to wait=u32 10) -> ()  [unwired: 1 out]
  }
  n139 = call "Attitude Control Close.vi"("Attitude Control Handle"=w1) -> ()  [unwired: 10 in, 1 out]
